vi "_058.vi"() -> ()   [LabVIEW 2024]
panel:
  out "Signals":dynamicdata(graph)
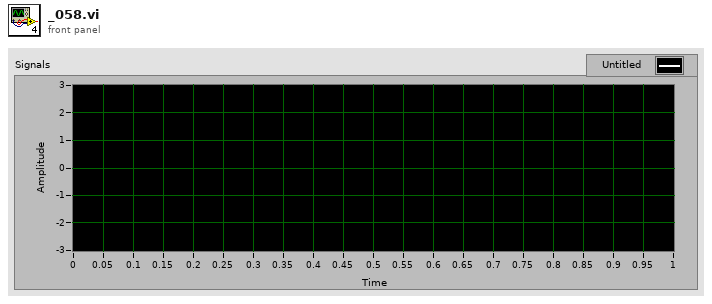
[diagram p1: front panel]
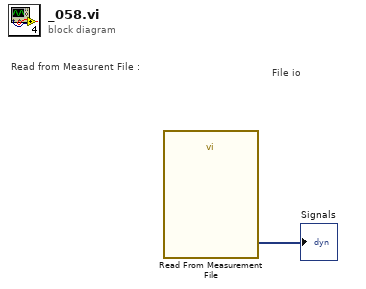
[diagram p0: block diagram]
diagram:
  # "File io"
  # "Read from Measurent File :"
  n1 = call "Read From Measurement File"() -> ("Signals"=→"Signals":dynamicdata)  [unwired: 6 in, 5 out]
